vi "Handle setConfiguration.vi"(8 "error in (no error)":errorcluster, 10 "setConfiguration":variant, 11 "Inst.Transport in":refnum<class "Inst.Transport.lvclass">) -> (0 "error out":errorcluster, 3 "Inst.Transport out":refnum<class "Inst.Transport.lvclass">)   [LabVIEW 2019, in "Inst.Transport.lvclass"]
uses:
  Inst.Transport.lvclass
  Inst.Transport.lvclass/Inst.Transport.ctl
  3f43cf47-96c4-42eb-930c-20be6e2d6ff8.vi
  3f43cf47-96c4-42eb-930c-20be6e2d6ff8.vi/416efcdc-ded0-4204-95af-3dc2b4e421c1.vi
  3f43cf47-96c4-42eb-930c-20be6e2d6ff8.vi/0ff53296-c4a9-4e04-bb3a-c685abebf105.vi
  <vilib>/Utility/Data Type/Get Type Information.vi
  <vilib>/JDP Science/JSONtext/JSON text to Variant.vi
  <vilib>/JDP Science/JSONtext/LVClass Serializer/JSONtext LVClass Serializer.lvclass
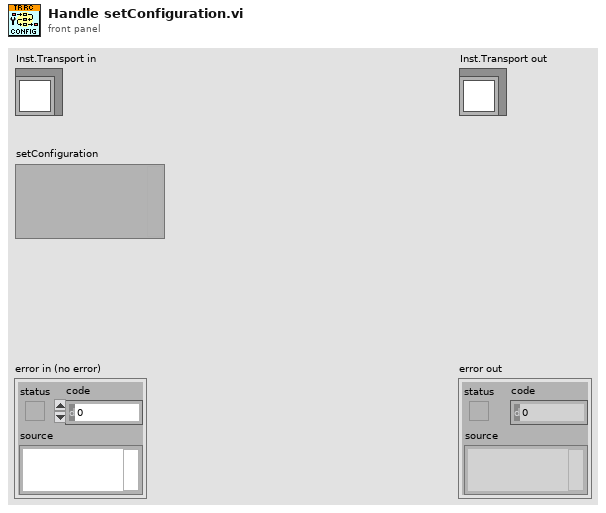
[diagram p1: front panel]
types:
  T1 = typedef "Inst.Transport.lvclass/Inst.Transport.Configuration--Cluster.ctl" = cluster{"Folder":string, "Comments":string}
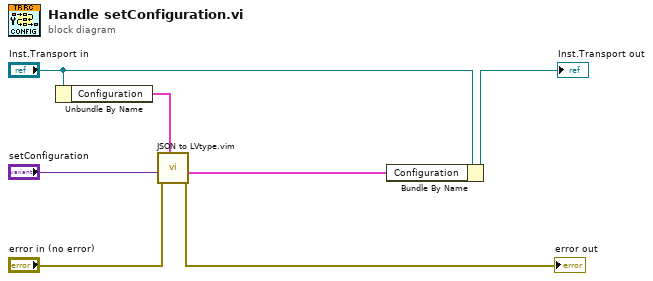
[diagram p0: block diagram]
diagram:
  n1 = Unbundle By Name("Inst.Transport in") -> ("Configuration"=w3:T1)
  n2 = call "JSON to LVtype.vim"("type"=w3, "error in (no error)"="error in (no error)", "JSON Data in"="setConfiguration") -> ("error out"=→"error out":errorcluster, "Data out"=w2:T1)  [unwired: 7 in]
  n3 = Bundle By Name(cluster="Inst.Transport in", "Configuration"=w2) -> (→"Inst.Transport out":refnum<class "Inst.Transport.lvclass">)
